vi "serial read.vi"() -> ()   [LabVIEW 2010]
uses:
  <vilib>/rvi/interface/nirviMethod/nirviMethod.xnode
  C:/Users/HAGAR-IV/Desktop/Zeugs/markus/version feb 2012/FPGA Bitfiles/pertrasgcfpga2_FPGATarget_FPGA-Programm-05_A75D3647.lvbitx
  C:/Users/HAGAR-IV/Desktop/Zeugs/Johnny/pertrasgc fpga/FPGA-Programm-05-17.vi
  <vilib>/rvi/interface/common/niFpgaNodeNameForErrorReporting.ctl
  <vilib>/rvi/errors/niLvFpgaWhatHappensToTopLevelVI.ctl
  <vilib>/rvi/interface/nirviReadWriteControl/nirviReadWriteControl.xnode
  <vilib>/rvi/interface/nirviCloseFPGA/nirviCloseFPGA.xnode
  <vilib>/Utility/error.llb/Error Cluster From Error Code.vi
  <vilib>/rvi/errors/niLvFpgaAdjustHostInterfaceError.vi
  <vilib>/FPGAPlugInAG/cRIO-9114/niLvFpga_Close_cRIO-9114.vi
  NiFpgaLv.dll
panel:
  in  "stop":bool
  out "concatenated string":string
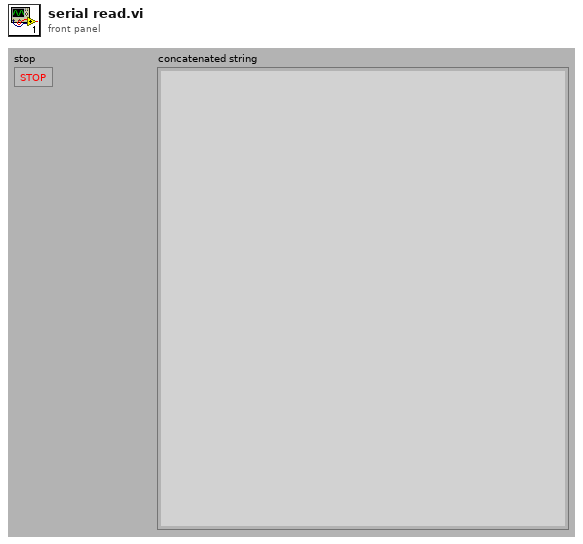
[diagram p1: front panel]
types:
  T1 = typedef "niFpgaNodeNameForErrorReporting.ctl" = enum16{"Open FPGA VI Reference", "Read/Write Control", "Invoke Method: Abort", "Invoke Method: Acknowledge IRQ", "Invoke Method: Download", "Invoke Method: FIFO.Configure", "Invoke Method: FIFO.Read", "Invoke Method: FIFO.Start", "Invoke Method: FIFO.Stop", "Invoke Method: FIFO.Write", "Invoke Method: Reset", "Invoke Method: Run", "Invoke Method: Wait on IRQ", "Close FPGA VI Reference"}
  T2 = typedef "niLvFpgaWhatHappensToTopLevelVI.ctl" = enum16{"top level VI scripted behind XNode", "top level VI inlined behind XNode"}
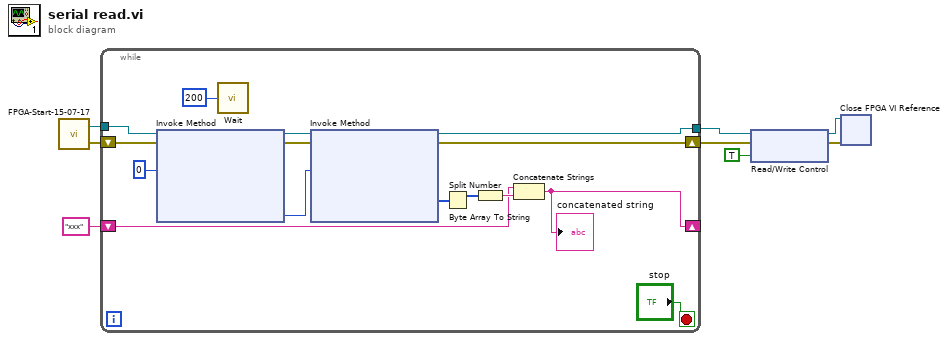
[diagram p0: block diagram]
diagram:
  n1 = call "FPGA-Start-15-07-17.vi"() -> ("error out"=w7:errorcluster, "FPGA VI Reference Out"=w8:refnum<k20>)  [unwired: 2 in]
  n2 = while {
    tunnel: w8 -> [w23]
    shift-right: [w17] -> w4
    shift-left: w7 -> [w20]
    shift-right: [w13] -> _
    shift-left: "xxx" -> [w12]
    tunnel: [w10] -> w5
    stop <- "stop" stop-if-true
    n3 = xnode "Invoke Method"("FPGA VI Reference In"=w23, "error in"=w20, "Number of Elements"=u32 0) -> ("FPGA VI Reference Out"=w18:refnum<k20>, "error out"=w19:errorcluster, "Elements Remaining"=w22:u32)  [unwired: 1 in, 1 out]
    n4 = call "Wait"("Count(mSec)"=u32 200) -> ()  [unwired: 1 out]
    n5 = xnode "Invoke Method"("FPGA VI Reference In"=w18, "error in"=w19, "Number of Elements"=w22) -> ("FPGA VI Reference Out"=w10:refnum<k20>, "error out"=w17:errorcluster, "Data"=w16:u16[])  [unwired: 1 in, 1 out]
    n6 = Split Number(x=w16) -> (hi(x)=w15:u8[])  [unwired: 1 out]
    n7 = Byte Array To String(unsigned byte array=w15) -> (string=w14:string)
    n8 = Concatenate Strings(w12, w14) -> (w13:string)
    "concatenated string" <- w13
  }
  n9 = xnode "Read/Write Control"("FPGA VI Reference In"=w5, "error in"=w4, "global stop"=TRUE) -> ("FPGA VI Reference Out"=w2:refnum<k20>, "error out"=w1:errorcluster)
  n10 = xnode "Close FPGA VI Reference"("FPGA VI Reference In"=w2, "error in"=w1) -> ()  [unwired: 1 out]
